vi "Facade ListBox.vi"(0 "Data In":T4, 2 "Display State In":T2, 3 "Container State":T3) -> (6 "Data Out":T4, 7 "Display State Out":T2, 8 "Action":T1)   [LabVIEW 2018, in "ListBox XControl.xctl"]
uses:
  ListBox XControl.xctl
  Data ListBox.ctl
  <vilib>/_xctls/Container State.ctl
  State ListBox.ctl
  <vilib>/_xctls/Action.ctl
  <vilib>/_xctls/XControlSupport.lvlib
panel:
  in  "Listbox":i32(listbox)
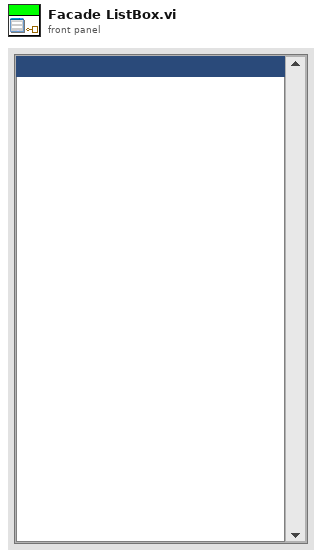
[diagram p1: front panel]
types:
  T1 = typedef "XControlSupport.lvlib/Action.ctl" = cluster{"Data Changed?":bool, "State Changed?":bool, "Action Name":string}
  T2 = typedef "ListBox XControl.xctl/State ListBox.ctl" = cluster{"ItemNames[]":string[], "Listbox Ref":refnum<vi>, "Select All By Default":bool}
  T3 = typedef "XControlSupport.lvlib/Container State.ctl" = cluster{"Indicator?":bool, "Run Mode?":bool, " Refnum":refnum<vi>}
  T4 = typedef "ListBox XControl.xctl/Data ListBox.ctl" = string[]
  T5 = typedef "LVPoint32TypeDef.ctl" = cluster{"Horizontal":i32, "Vertical":i32}
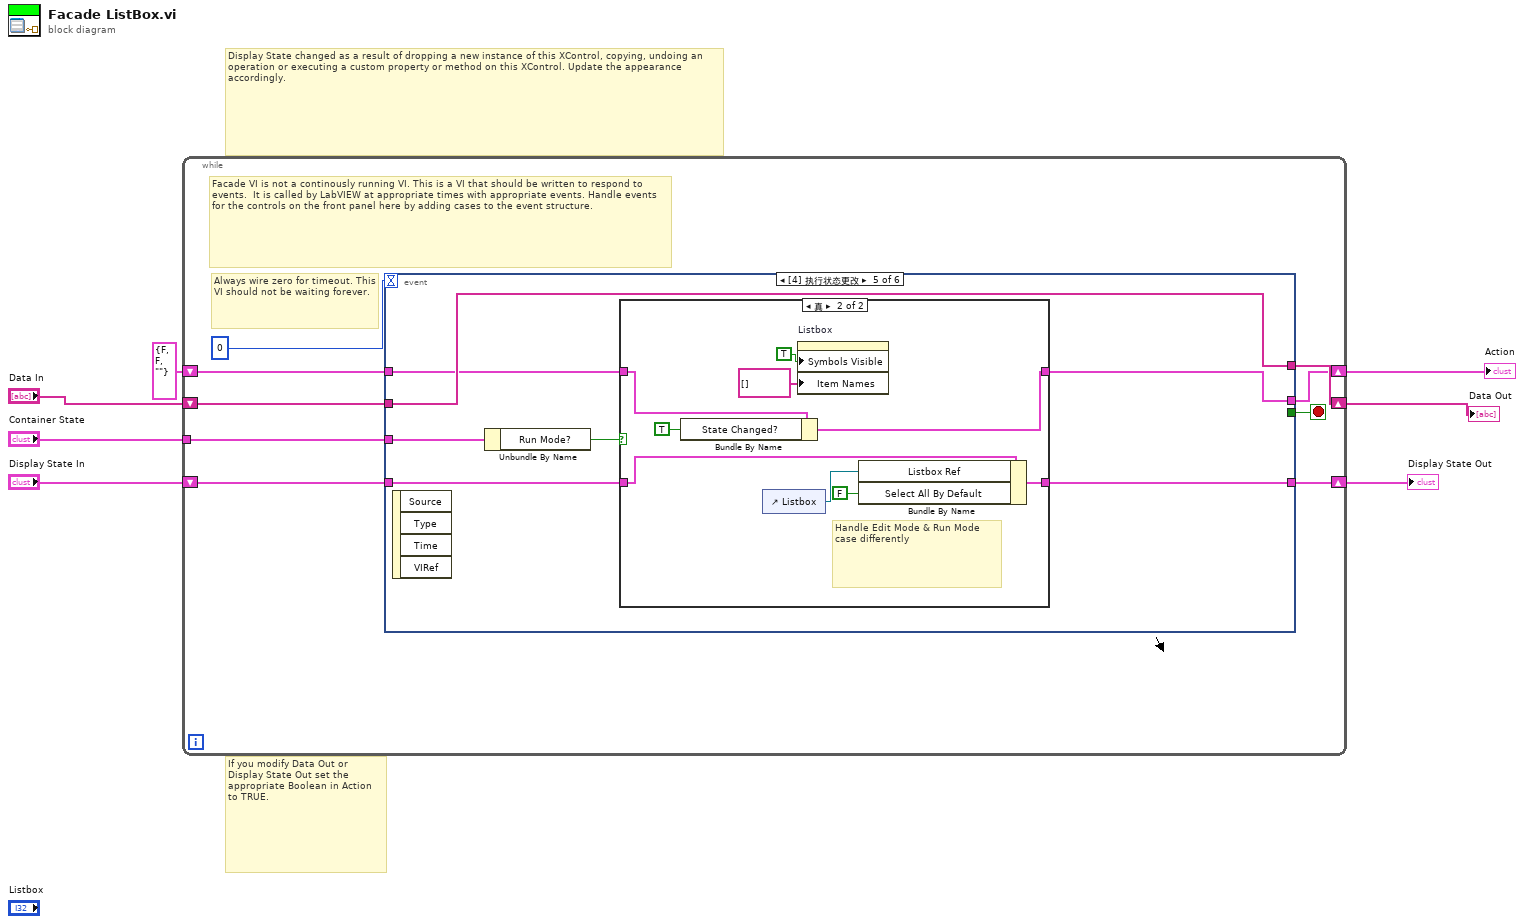
[diagram p0: block diagram]
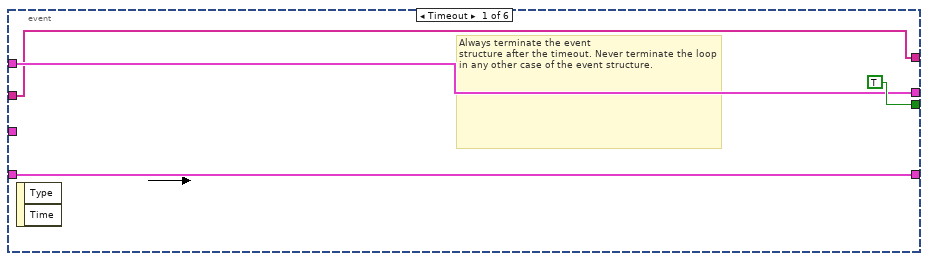
[diagram p2: hidden frame]
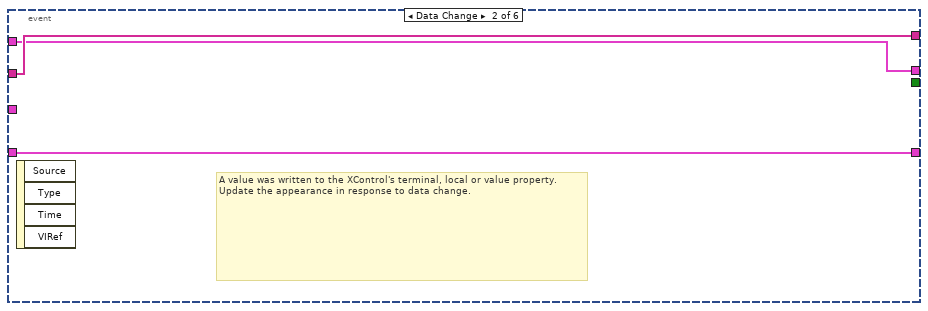
[diagram p3: hidden frame]
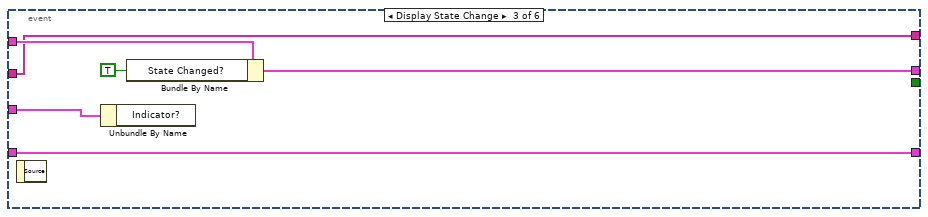
[diagram p4: hidden frame]
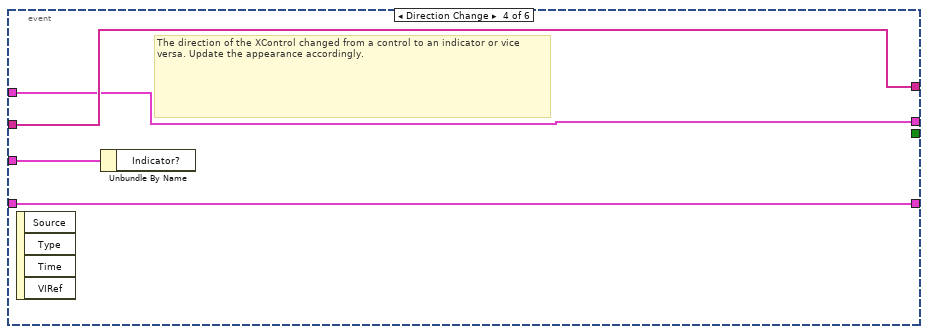
[diagram p5: hidden frame]
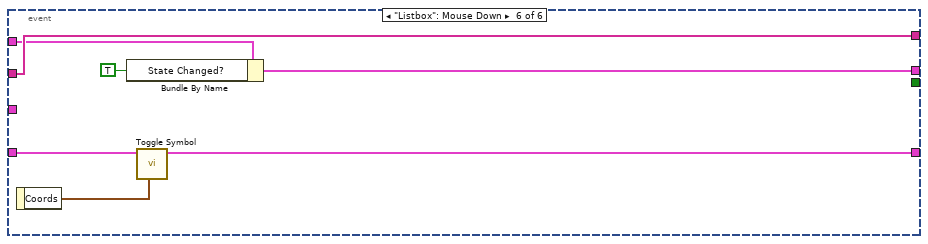
[diagram p7: hidden frame]
diagram:
  # "Display State changed as a result of dropping a new instance of this XControl, copying, undoing an operation or executing a custom property or method on this XControl. Update the appearance accordingly."
  # "If you modify Data Out or\nDisplay State Out set the\nappropriate Boolean in Action\nto TRUE."
  n1 = while {
    shift-right: [w15] -> w4
    shift-left: "Display State In" -> [w16]
    tunnel: "Container State" -> [w12]
    shift-right: [w10] -> w7
    shift-left: "Data In" -> [w11]
    shift-right: [w8] -> w2
    shift-left: T1 {"Data Changed?"=FALSE, "State Changed?"=FALSE, "Action Name"=""} ("Action") -> [w9]
    stop <- w14 stop-if-true
    # "Facade VI is not a continously running VI. This is a VI that should be written to respond to events.  It is called by LabVIEW at appropriate times with appropriate events. Handle events for the controls on the front panel here by adding cases to the event structure."
    # "Always wire zero for timeout. This\nVI should not be waiting forever."
    n2 = event shown="[4] 执行状态更改" {
      selector: _ -> [_ _ _ _ _ _]
      dyn-events: _ -> [_ _ _ _ _ _]
      timeout: 0 -> [_ _ _ _ _ _]
      tunnel: w16 -> [w18 w22 w25 w32 w37 w54]
      tunnel: [w18 w22 w25 w32 w36 w53] -> w15
      tunnel: [TRUE _ _ _ _ _] -> w14
      tunnel: w12 -> [_ _ w24 w33 w40 _]
      tunnel: w11 -> [w17 w23 w28 w31 w39 w58]
      tunnel: [w17 w23 w28 w31 w39 w58] -> w10
      tunnel: [w19 w21 w27 w30 w35 w56] -> w8
      tunnel: w9 -> [w19 w21 w29 w30 w38 w57]
      event Timeout {
        # "Always terminate the event\nstructure after the timeout. Never terminate the loop in any other case of the event structure."
        n3 = event-data() -> ()  [unwired: 1 in, 2 out]
      }
      event Data Change {
        # "A value was written to the XControl's terminal, local or value property.\nUpdate the appearance in response to data change."
        n4 = event-data() -> ()  [unwired: 1 in, 4 out]
      }
      event Display State Change {
        n5 = event-data() -> ()  [unwired: 1 in, 1 out]
        n6 = Unbundle By Name(w24) -> ()  [unwired: 1 out]
        n7 = Bundle By Name(cluster=w29, "State Changed?"=TRUE ("Data Changed?")) -> (w27:T1)
      }
      event Direction Change {
        # "The direction of the XControl changed from a control to an indicator or vice versa. Update the appearance accordingly."
        n8 = event-data() -> ()  [unwired: 1 in, 4 out]
        n9 = Unbundle By Name(w33) -> ()  [unwired: 1 out]
      }
      event Exec State Change {
        n10 = event-data() -> ()  [unwired: 1 in, 4 out]
        n11 = Unbundle By Name(w40) -> ("Run Mode?"=w34:bool)
        n12 = case shown="真" w34 {
          tunnel: w38 -> [w41 w51]
          tunnel: w37 -> [w42 w47]
          tunnel: [w42 w46] -> w36
          tunnel: [w41 w45] -> w35
          frame False {
          }
          frame True {
            # "Handle Edit Mode & Run Mode\ncase differently"
            n13 = Bundle By Name(cluster=w51, "State Changed?"=TRUE) -> (w45:T1)
            n14 = control-ref of="Listbox"() -> (w48:refnum<vi>)
            n15 = property on="Listbox" class="LstBox (严格)"("Symbols Visible"=TRUE ("Visible Items:Symbols Visible"), "Item Names"=string[] []) -> ()  [unwired: 2 in, 2 out]
            n16 = Bundle By Name(cluster=w47, "Listbox Ref"=w48, "Select All By Default"=FALSE) -> (w46:T2)
          }
        }
      }
      event "Listbox": Mouse Down {
        n17 = event-data() -> ("Coords"=w52:T5)  [unwired: 1 in]
        n18 = Bundle By Name(cluster=w57, "State Changed?"=TRUE) -> (w56:T1)
        n19 = call "Toggle Symbol.vi"("Coords"=w52, "Display State In"=w54) -> ("Display State In 2"=w53:T2)  [unwired: 9 in]
      }
    }
  }
  "Display State Out" <- w4
  "Data Out" <- w7
  "Action" <- w2
